vi "MotorControl.vi"(0 "Ring":u16(ring) items=["Horizontal", "Vertical"], 1 "Direction":bool=TRUE, 2 "Step rate":dbl, 3 "number of steps":i32=1000, 4 "error in":errorcluster) -> (5 "error out":errorcluster)   [LabVIEW 2018]
uses:
  <vilib>/DAQmx/write.llb/DAQmx Write (Digital Bool 1Line 1Point).vi
  <vilib>/DAQmx/write.llb/DAQmx Write (Digital 1D U32 1Chan NSamp).vi
  <vilib>/DAQmx/create/channels.llb/DAQmx Create Channel (DO-Digital Output).vi
  <vilib>/DAQmx/miscellaneous.llb/DAQmx Fill In Error Info.vi
  <vilib>/DAQmx/create/channels.llb/DAQmx Create Channel (CO-Pulse Generation-Frequency).vi
  <vilib>/DAQmx/configure/timing.llb/DAQmx Timing (Implicit).vi
  <vilib>/DAQmx/configure/timing.llb/DAQmx Timing (Sample Clock).vi
panel:
  in  "rate":dbl=1000.0 format="%0.2f"
  out "error out 2":errorcluster
  in  "stop":bool
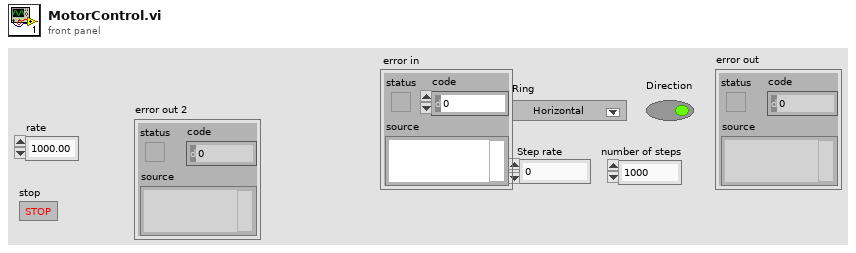
[diagram p1: front panel]
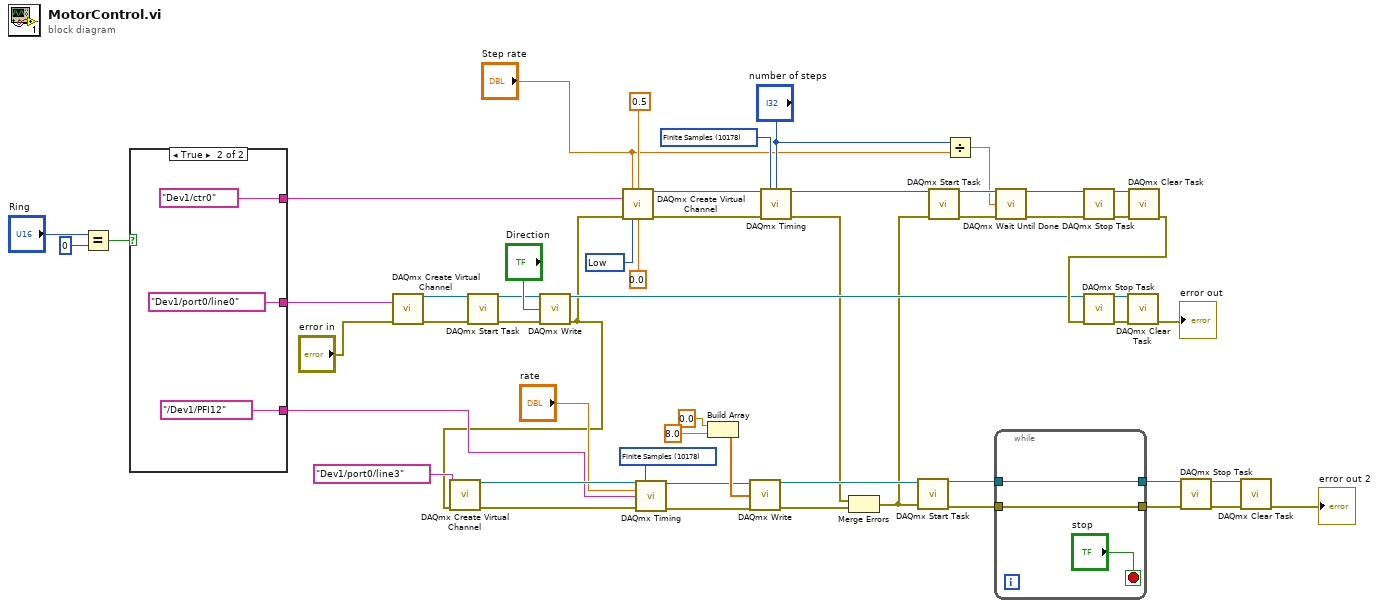
[diagram p0: block diagram]
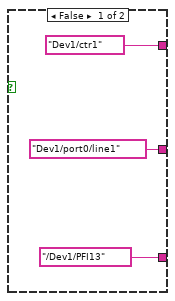
[diagram p2: hidden frame]
diagram:
  w19 = 10178 items=["Finite Samples"=10178, "Continuous Samples"=10123, "Hardware Timed Single Point"=12522] ("sample mode")
  w48 = 10214 items=["High"=10192, "Low"=10214] ("idle state")
  w55 = 10178 items=["Finite Samples"=10178, "Continuous Samples"=10123, "Hardware Timed Single Point"=12522] ("sample mode")
  n1 = Equal?(x="Ring", y=u16 0) -> (x = y?=w52:bool)
  n2 = case shown="True" w52 {
    tunnel: [tag "Dev1/ctr1" ("counter") tag "Dev1/ctr0" ("counter")] -> w46
    tunnel: [tag "Dev1/port0/line1" ("lines") tag "Dev1/port0/line0" ("lines")] -> w45
    tunnel: [tag "/Dev1/PFI13" ("source") tag "/Dev1/PFI12" ("source")] -> w5
    frame False {
    }
    frame True {
    }
  }
  n3 = call-poly <vilib>:"DAQmx Create Virtual Channel.vi"("lines"=w45, "error in"="error in") -> ("task out"=w44:refnum<k21>, "error out"=w43:errorcluster)  [unwired: 12 in]
  n4 = call <vilib>:"DAQmx Start Task.vi"("task/channels in"=w44, "error in"=w43) -> ("task out"=w41:refnum<k21>, "error out"=w40:errorcluster)  [unwired: 12 in]
  n5 = call-poly <vilib>:"DAQmx Write.vi"("task/channels in"=w41, "data"="Direction", "error in"=w40) -> ("task out"=w27:refnum<k21>, "error out"=w4:errorcluster)  [unwired: 10 in, 1 out]
  n6 = call-poly <vilib>:"DAQmx Create Virtual Channel.vi"("lines"=tag "Dev1/port0/line3", "error in"=w4) -> ("task out"=w18:refnum<k21>, "error out"=w17:errorcluster)  [unwired: 12 in]
  n7 = call-poly <vilib>:"DAQmx Create Virtual Channel.vi"("frequency"="Step rate", "duty cycle"=0.5, "counter"=w46, "error in"=w4, "idle state"=w48, "initial delay"=0.0) -> ("task out"=w32:refnum<k21>, "error out"=w31:errorcluster)  [unwired: 8 in]
  n8 = call-poly <vilib>:"DAQmx Timing.vi"("task/channels in"=w18, "sample mode"=w19, "rate"="rate", "source"=w5, "error in"=w17) -> ("task out"=w12:refnum<k21>, "error out"=w11:errorcluster)  [unwired: 9 in]
  n9 = Build Array(0.0 ("element"), 8.0 ("element")) -> (w14:dbl[])
  n10 = call-poly <vilib>:"DAQmx Write.vi"("task/channels in"=w12, "data"=w14, "error in"=w11) -> ("task out"=w10:refnum<k21>, "error out"=w2:errorcluster)  [unwired: 10 in, 1 out]
  n11 = call-poly <vilib>:"DAQmx Timing.vi"("task/channels in"=w32, "sample mode"=w55, "samples per channel"="number of steps", "error in"=w31) -> ("task out"=w50:refnum<k21>, "error out"=w3:errorcluster)  [unwired: 10 in]
  n12 = Merge Errors(w3, w2) -> (w1:errorcluster)
  n13 = call <vilib>:"DAQmx Start Task.vi"("task/channels in"=w10, "error in"=w1) -> ("task out"=w9:refnum<k21>, "error out"=w8:errorcluster)  [unwired: 12 in]
  n14 = call <vilib>:"DAQmx Start Task.vi"("task/channels in"=w50, "error in"=w1) -> ("task out"=w30:refnum<k21>, "error out"=w47:errorcluster)  [unwired: 12 in]
  n15 = Divide(x="number of steps", y="Step rate") -> (x/y=w28:dbl)
  n16 = while {
    tunnel: w9 -> [w63]
    tunnel: [w63] -> w16
    tunnel: [w62] -> w15
    tunnel: w8 -> [w62]
    stop <- "stop" stop-if-true
  }
  n17 = call <vilib>:"DAQmx Wait Until Done.vi"("task/channels in"=w30, "timeout (sec)"=w28, "error in"=w47) -> ("task out"=w37:refnum<k21>, "error out"=w35:errorcluster)  [unwired: 11 in]
  n18 = call <vilib>:"DAQmx Stop Task.vi"("task/channels in"=w37, "error in"=w35) -> ("task out"=w49:refnum<k21>, "error out"=w34:errorcluster)  [unwired: 12 in]
  n19 = call <vilib>:"DAQmx Clear Task.vi"("task in"=w49, "error in"=w34) -> ("error out"=w33:errorcluster)  [unwired: 13 in]
  n20 = call <vilib>:"DAQmx Stop Task.vi"("task/channels in"=w27, "error in"=w33) -> ("task out"=w39:refnum<k21>, "error out"=w38:errorcluster)  [unwired: 12 in]
  n21 = call <vilib>:"DAQmx Clear Task.vi"("task in"=w39, "error in"=w38) -> ("error out"=→"error out":errorcluster)  [unwired: 13 in]
  n22 = call <vilib>:"DAQmx Stop Task.vi"("task/channels in"=w16, "error in"=w15) -> ("task out"=w23:refnum<k21>, "error out"=w22:errorcluster)  [unwired: 12 in]
  n23 = call <vilib>:"DAQmx Clear Task.vi"("task in"=w23, "error in"=w22) -> ("error out"=→"error out 2":errorcluster)  [unwired: 13 in]
